vi "Store Instrument State.vi"(8 "error in (no error)":errorcluster, 9 "Items (3: CDState)":u16(ring)=3 items=["State", "CState", "Dstate", "CDState"], 10 "Store All Channels/Traces (F:  Displayed Channels/traces Only)":bool, 11 "VISA resource name":refnum<visa-resource-name>) -> (0 "error out":errorcluster, 3 "VISA resource name out":refnum<visa-resource-name>)   [LabVIEW 2022 SP3, in "Agilent ENA Series.lvlib"]
doc: "Configures file handling.\n\n<b>Note:</b>\nThe E5080A and E5080B only supports saving the displayed channels/traces only."
uses:
  <instrlib>/Agilent ENA Series/Agilent ENA Series.lvlib
panel:
  # "Note:\nThe E5080A and E5080B only supports saving the displayed channels/traces only."
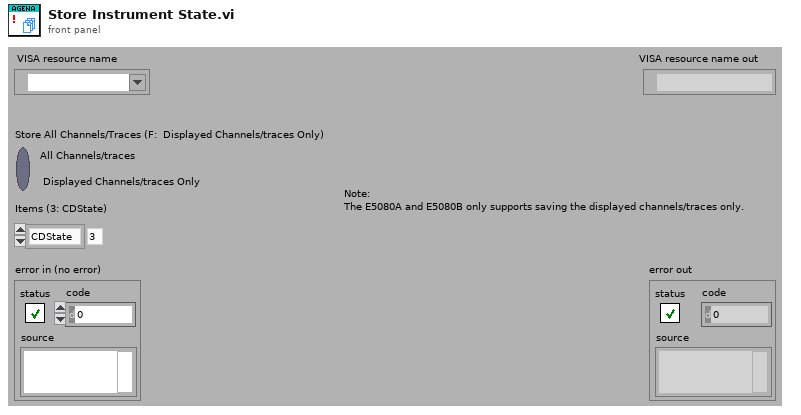
[diagram p1: front panel]
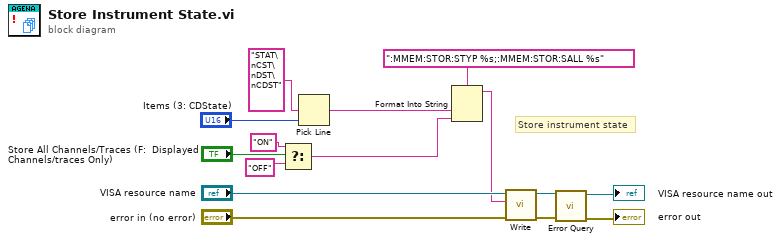
[diagram p0: block diagram]
diagram:
  # "Store instrument state"
  n1 = Select(t="ON", s="Store All Channels/Traces (F:  Displayed Channels/traces Only)", f="OFF") -> (s? t:f=w6:string)
  n2 = Pick Line(multi-line string="STAT\nCST\nDST\nCDST", line index="Items (3: CDState)") -> (output string=w11:string)  [unwired: 1 in]
  n3 = Format Into String(format string=":MMEM:STOR:STYP %s;:MMEM:STOR:SALL %s", w11, w6) -> (resulting string=w7:string)  [unwired: 2 in, 1 out]
  n4 = call <instrlib>:"Write.vi"("error in (no error)"="error in (no error)", "String ()"=w7, "VISA resource name"="VISA resource name") -> ("error out"=w3:errorcluster, "VISA resource name out"=w4:refnum<visa-resource-name>)  [unwired: 6 in, 1 out]
  n5 = call <instrlib>:"Error Query.vi"("error in (no error)"=w3, "VISA resource name"=w4) -> ("error out"=→"error out":errorcluster, "VISA resource name out"=→"VISA resource name out":refnum<visa-resource-name>)  [unwired: 6 in, 2 out]
